vi "1D DBL To String Array.vi"(10 "Array In":dbl[](array[numeric]) format="%#_f") -> (2 "String Array Out":string[](array[string]))   [LabVIEW 2024]
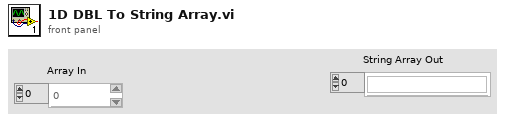
[diagram p1: front panel]
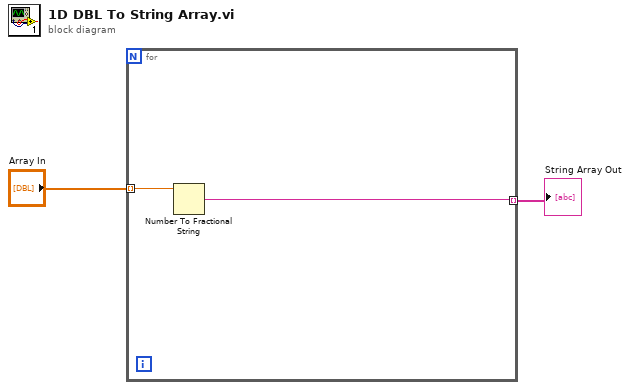
[diagram p0: block diagram]
diagram:
  n1 = for {
    tunnel: "Array In" -> [w4] mode=indexing
    tunnel: [w3] -> w1 mode=indexing
    n2 = Number To Fractional String(number=w4) -> (F-format string=w3:string)  [unwired: 3 in]
  }
  "String Array Out" <- w1
